vi "Configure Arbitrary Waveform.vi"(4 "Frequency (1000 Hz)":dbl=1000.0, 5 "File Path":string, 6 "DC Offset (0 V)":dbl, 7 "Arbitrary Waveform Name (0: USER1)":u16(ring) items=["USER1", "USER2", "USER3", "USER4", "Edit Memory", "Edit Path"], 8 "error in (no error)":errorcluster, 9 "Gain (1 V)":dbl=1.0, 10 "Channel (0: Channel 1)":u16(ring) items=["Channel 1", "Channel 2"], 11 "VISA resource name":refnum<visa-resource-name>) -> (0 "error out":errorcluster, 3 "VISA resource name out":refnum<visa-resource-name>)   [LabVIEW 2015, in "Tektronix AFG 3000 Series.lvlib"]
doc: "Configures the function generator settings that affect arbitrary waveform generation."
uses:
  Tektronix AFG 3000 Series.lvlib
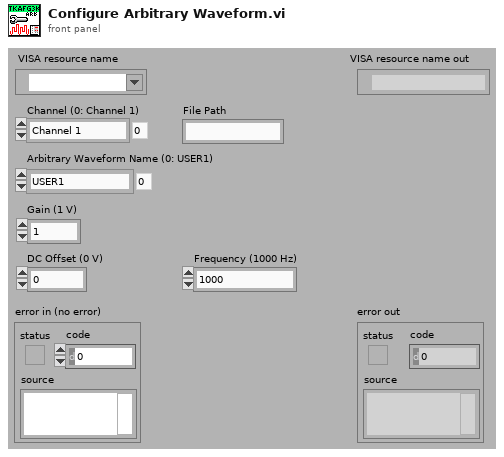
[diagram p1: front panel]
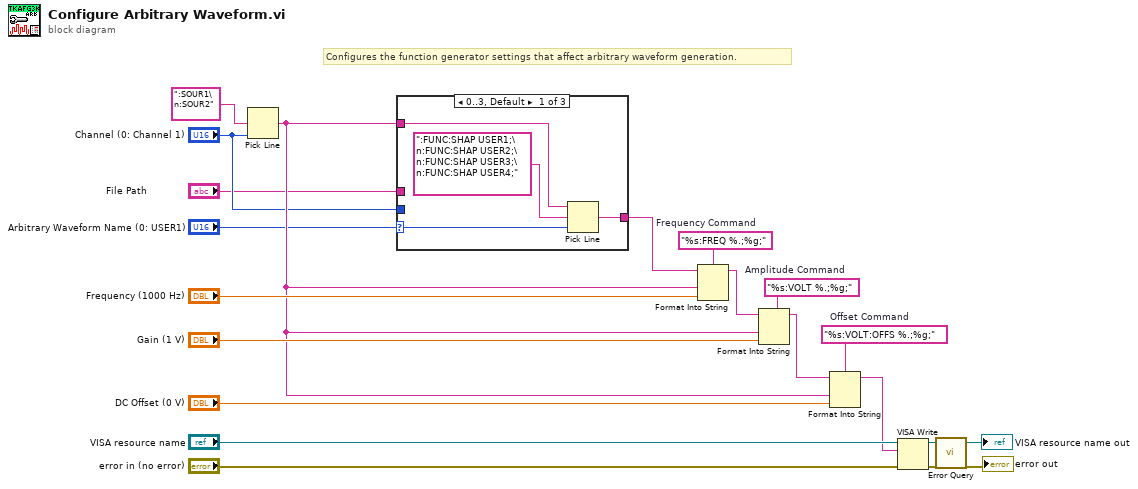
[diagram p0: block diagram]
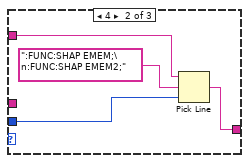
[diagram p2: hidden frame]
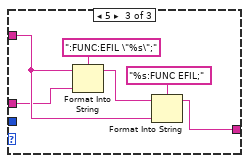
[diagram p3: hidden frame]
diagram:
  w8 = "%s:VOLT:OFFS %.;%g;"  # Offset Command
  w9 = "%s:VOLT %.;%g;"  # Amplitude Command
  w10 = "%s:FREQ %.;%g;"  # Frequency Command
  # "Configures the function generator settings that affect arbitrary waveform generation."
  n1 = Pick Line(multi-line string=":SOUR1\n:SOUR2" ("string (\"\")"), line index="Channel (0: Channel 1)") -> (output string=w4:string)  [unwired: 1 in]
  n2 = case shown="0..3, Default" "Arbitrary Waveform Name (0: USER1)" {
    selector: "Arbitrary Waveform Name (0: USER1)" -> [w23 _ _]
    tunnel: [w22 w26 w30] -> w11
    tunnel: w4 -> [w25 w29 w32]
    tunnel: "Channel (0: Channel 1)" -> [_ w27 _]
    tunnel: "File Path" -> [_ _ w31]
    frame 0..3, Default {
      n3 = Pick Line(string ("")=w25, multi-line string=":FUNC:SHAP USER1;\n:FUNC:SHAP USER2;\n:FUNC:SHAP USER3;\n:FUNC:SHAP USER4;" ("string (\"\")"), line index=w23) -> (output string=w22:string)
    }
    frame 4 {
      n4 = Pick Line(string ("")=w29, multi-line string=":FUNC:SHAP EMEM;\n:FUNC:SHAP EMEM2;" ("string (\"\")"), line index=w27) -> (output string=w26:string)
    }
    frame 5 {
      n5 = Format Into String(format string=":FUNC:EFIL \"%s\";", initial string=w32, w31) -> (resulting string=w34:string)  [unwired: 1 in, 1 out]
      n6 = Format Into String(format string="%s:FUNC EFIL;", initial string=w34, w32) -> (resulting string=w30:string)  [unwired: 1 in, 1 out]
    }
  }
  n7 = Format Into String(format string=w10, initial string=w11, w4, "Frequency (1000 Hz)") -> (resulting string=w13:string)  [unwired: 1 in, 1 out]
  n8 = Format Into String(format string=w9, initial string=w13, w4, "Gain (1 V)") -> (resulting string=w12:string)  [unwired: 1 in, 1 out]
  n9 = Format Into String(format string=w8, initial string=w12, w4, "DC Offset (0 V)") -> (resulting string=w15:string)  [unwired: 1 in, 1 out]
  n10 = VISA Write(VISA resource name="VISA resource name", write buffer=w15, error in (no error)="error in (no error)") -> (VISA resource name out=w19:refnum<visa-resource-name>, error out=w18:errorcluster)  [unwired: 1 out]
  n11 = call "Error Query.vi"("error in (no error)"=w18, "VISA resource name"=w19) -> ("error out"=→"error out":errorcluster, "VISA resource name out"=→"VISA resource name out":refnum<visa-resource-name>)  [unwired: 6 in, 2 out]
